vi "TurnToAngleController.vi"(0 "TargetAngle":dbl=600.0, 1 "MaxVel":dbl=80.0, 3 "MaxAccel":dbl=150.0, 5 "Robot":T1={"Angle"=548.1299999999924, "Angular vel"=0.49263510517714687, "Left Distance"=26.0882735, "Left vel"=0.0, "Right Distance"=-234.57467250000002, "Right vel"=0.0}, 9 "Gains":T2={"Gains"={"FFV"=0.0061, "FFA"=0.0024, "Vel PID"={"P"=0.0, "I"=0.0, "D"=0.0}}, "Pos PID"={"P"=0.0, "I"=0.0, "D"=0.0}, "MinVoltage"=0.25, "Effective Trackwidth"=30.0, "Effective Trackwidth CCW"=30.0} {"Pos PID"."D" format="%.3f"; "Pos PID"."I" format="%.3f"; "Pos PID"."P" format="%.3f"; "Gains"."Vel PID"."D" format="%.3f"; "Gains"."Vel PID"."I" format="%.3f"; "Gains"."Vel PID"."P" format="%.3f"}, 11 "Reset":bool, 13 "GoSmallestDistance":bool) -> (4 "LeftPower":dbl=0.25, 6 "RightPower":dbl=-0.25, 8 "Encoder Distance":cluster{"Output":dbl, "dx/dt":dbl}(graph)={"Output"=52.36486996421861, "dx/dt"=26.0882735}, 10 "Delay":dbl=20.0, 12 "Angle":cluster{"Distance":dbl, "CurrentAngle":dbl}(graph)={"Distance"=-120.0, "CurrentAngle"=-171.87000000000762}, 14 "VelGraph":cluster{"Output":dbl, "dx/dt":dbl}(graph), 15 "Done":bool)   [LabVIEW 2018]
uses:
  <vilib>/addons/control/pid/pid.llb/PID (DBL).vi
  <vilib>/addons/control/pid/NI_PID_pid.lvlib
panel:
  in  "Target Vel":dbl
  out "Power":dbl(graph)=0.25
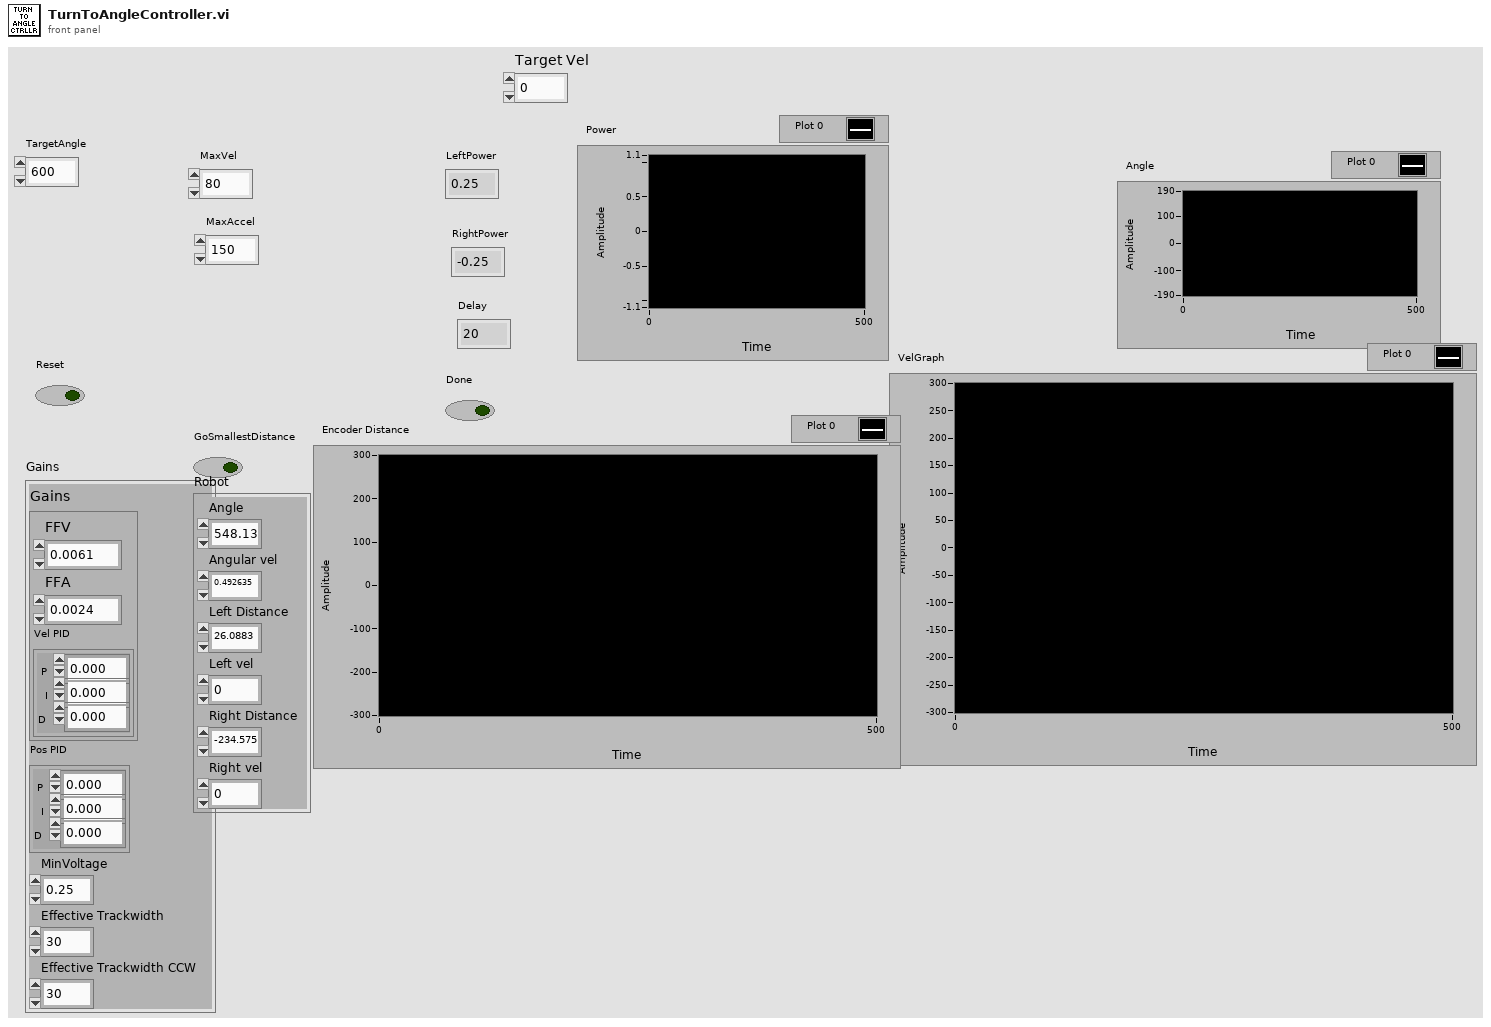
[diagram p1: front panel]
types:
  T1 = cluster{"Angle":dbl, "Angular vel":dbl, "Left Distance":dbl, "Left vel":dbl, "Right Distance":dbl, "Right vel":dbl}
  T2 = cluster{"Gains":cluster{"FFV":dbl, "FFA":dbl, "Vel PID":cluster{"P":dbl, "I":dbl, "D":dbl}}, "Pos PID":cluster{"P":dbl, "I":dbl, "D":dbl}, "MinVoltage":dbl, "Effective Trackwidth":dbl, "Effective Trackwidth CCW":dbl}
  T3 = cluster{"TargetPos":dbl, "InitalPos":dbl, "FinalVel":dbl, "IntitialVel":dbl, "MaxVel":dbl, "MaxAccel":dbl}
  T4 = cluster{"Smallest A to B":dbl, "Smallest A to B":dbl}
  T5 = cluster{"Smallest A to B":dbl, "Left Distance":dbl}
  T6 = cluster{"FFV":dbl, "FFA":dbl, "Vel PID":cluster{"P":dbl, "I":dbl, "D":dbl}}
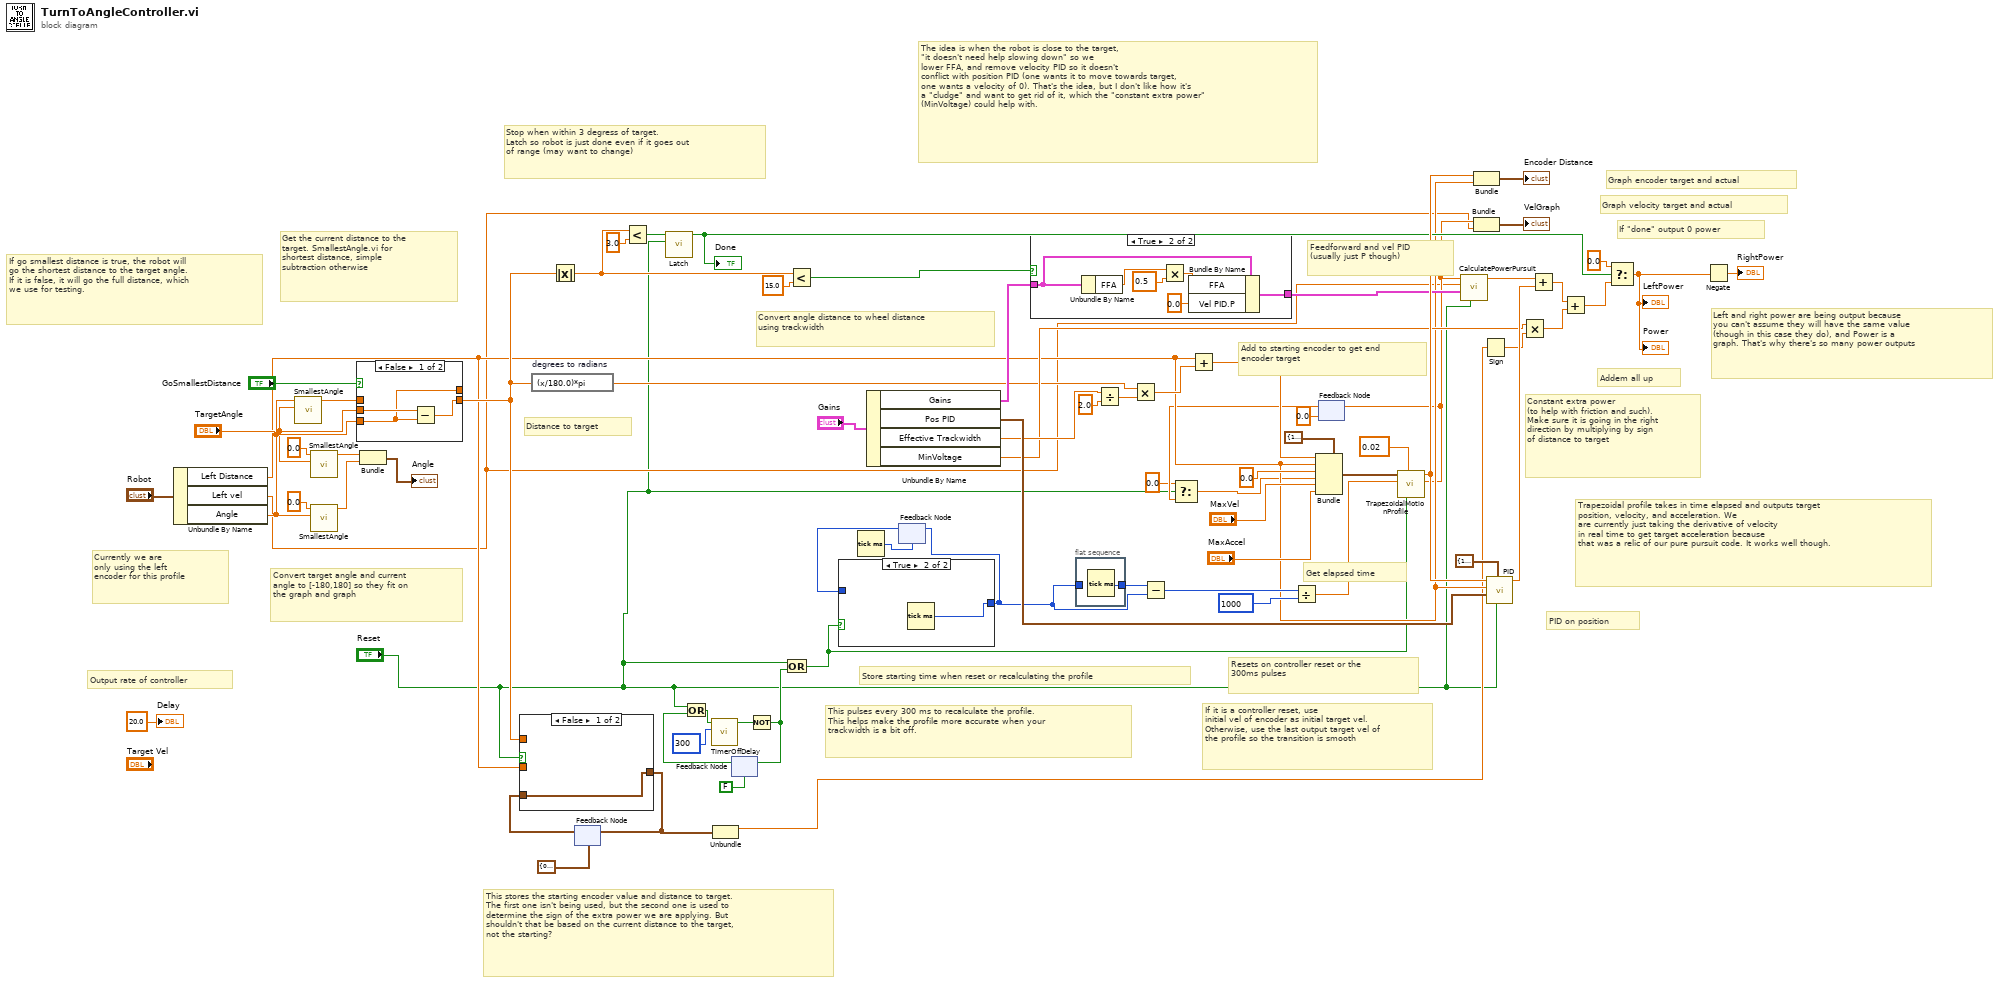
[diagram p0: block diagram]
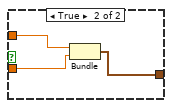
[diagram p2: hidden frame]
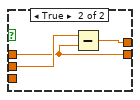
[diagram p4: hidden frame]
diagram:
  # "Currently we are\nonly using the left\nencoder for this profile"
  # "Output rate of controller"
  # "Addem all up"
  # "Left and right power are being output because\nyou can't assume they will have the same value\n(though in this case they do), and Power is a\ngraph. That's why there's so many power outputs"
  # "If \"done\" output 0 power"
  # "Graph velocity target and actual"
  # "Graph encoder target and actual"
  # "Feedforward and vel PID\n(usually just P though)"
  # "If it is a controller reset, use\ninitial vel of encoder as initial target vel.\nOtherwise, use the last output target vel of\nthe profile so the transition is smooth"
  # "Resets on controller reset or the \n300ms pulses"
  # "Trapezoidal profile takes in time elapsed and outputs target\nposition, velocity, and acceleration. We\nare currently just taking the derivative of velocity\nin real time to get target acceleration because\nthat was a relic of our pure pursuit code. It works well though."
  # "The idea is when the robot is close to the target,\n\"it doesn't need help slowing down\" so we\nlower FFA, and remove velocity PID so it doesn't\nconflict with position PID (one wants it to move towards target,\none wants a velocity of 0). That's the idea, but I don't like how it's\na \"cludge\" and want to get rid of it, which the \"constant extra power\"\n(MinVoltage) could help with."
  # "Add to starting encoder to get end\nencoder target"
  # "Convert angle distance to wheel distance\nusing trackwidth"
  # "Constant extra power\n(to help with friction and such).\nMake sure it is going in the right\ndirection by multiplying by sign\nof distance to target"
  # "PID on position"
  # "Get elapsed time"
  # "Store starting time when reset or recalculating the profile"
  # "This pulses every 300 ms to recalculate the profile.\nThis helps make the profile more accurate when your\ntrackwidth is a bit off."
  # "This stores the starting encoder value and distance to target.\nThe first one isn't being used, but the second one is used to\ndetermine the sign of the extra power we are applying. But\nshouldn't that be based on the current distance to the target,\nnot the starting?"
  # "Stop when within 3 degress of target.\nLatch so robot is just done even if it goes out\nof range (may want to change)"
  # "Get the current distance to the\ntarget. SmallestAngle.vi for \nshortest distance, simple\nsubtraction otherwise"
  # "If go smallest distance is true, the robot will\ngo the shortest distance to the target angle.\nIf it is false, it will go the full distance, which\nwe use for testing."
  # "Convert target angle and current\nangle to [-180,180] so they fit on\nthe graph and graph"
  # "Distance to target"
  n1 = Unbundle By Name("Robot") -> ("Left Distance"=w19:dbl, "Left vel"=w4:dbl, "Angle"=w53:dbl)
  n2 = call "SmallestAngle.vi"("Angle B"="TargetAngle", "Angle A"=w53) -> ("Smallest A to B"=w61:dbl)  [unwired: 9 in]
  n3 = call "SmallestAngle.vi"("Angle B"="TargetAngle", "Angle A"=0.0) -> ("Smallest A to B"=w51:dbl)  [unwired: 9 in]
  n4 = call "SmallestAngle.vi"("Angle B"=w53, "Angle A"=0.0) -> ("Smallest A to B"=w50:dbl)  [unwired: 9 in]
  n5 = case shown="False" "GoSmallestDistance" {
    tunnel: [w76 w80] -> _
    tunnel: "TargetAngle" -> [w77 w79]
    tunnel: w61 -> [_ w78]
    tunnel: [w75 w78] -> w20
    tunnel: w53 -> [w76 _]
    frame False {
      n6 = Subtract(x=w77, y=w76) -> (x-y=w75:dbl)
    }
    frame True {
      n7 = Subtract(x=w79, y=w78) -> (x-y=w80:dbl)
    }
  }
  n8 = Bundle("Smallest A to B"=w51, "Smallest A to B"=w50) -> (→"Angle":T4)  [unwired: 1 in]
  n9 = expression code="(x/180.0)*pi" "degrees to radians"(w20) -> (w18:dbl)
  n10 = Absolute Value(x=w20) -> (abs(x)=w31:dbl)
  n11 = feedback #1(cluster{"Angle":dbl, "Distance":dbl} {"Angle"=0.0, "Distance"=0.0}) -> (w35:cluster{"Angle":dbl, "Distance":dbl})
  n12 = case shown="False" "Reset" {
    tunnel: w20 -> [_ w84]
    tunnel: [w81 w83] -> w17
    tunnel: w35 -> [w81 _]
    tunnel: w19 -> [_ w82]
    frame False {
    }
    frame True {
      n13 = Bundle("Smallest A to B"=w84, "Left Distance"=w82) -> (w83:T5)  [unwired: 1 in]
    }
  }
  n14 = feedback-in #1(w17) -> ()
  n15 = Less?(x=w31, y=3.0) -> (x < y?=w57:bool)
  n16 = call "Latch.vi"("Reset"="Reset", "Input"=w57) -> ("Output"=w23:bool)  [unwired: 9 in]
  "Done" <- w23
  n17 = Unbundle(w17) -> ("Smallest A to B"=w16:dbl)  [unwired: 1 out]
  n18 = feedback #2(FALSE) -> (w11:bool)
  n19 = Or(x="Reset", y=w11) -> (x .or. y?=w12:bool)
  n20 = call "TimerOffDelay.vi"("Time Delay"=u32 300, "Input"=w12) -> ("Output"=w10:bool)  [unwired: 9 in]
  n21 = Not(x=w10) -> (.not. x?=w8:bool)
  n22 = feedback-in #2(w8) -> ()
  n23 = Or(x="Reset", y=w8) -> (x .or. y?=w14:bool)
  n24 = Less?(x=w31, y=15.0) -> (x < y?=w38:bool)
  n25 = Tick Count (ms)() -> (millisecond timer value=w36:u32)
  n26 = Unbundle By Name("Gains") -> ("Gains"=w39:T6, "Pos PID"=w45:cluster{"P":dbl, "I":dbl, "D":dbl}, "Effective Trackwidth"=w34:dbl, "MinVoltage"=w24:dbl)
  n27 = feedback #3(w36) -> (w37:u32)
  n28 = case shown="True" w14 {
    tunnel: [w85 w86] -> w29
    tunnel: w37 -> [w85 _]
    frame False {
    }
    frame True {
      n29 = Tick Count (ms)() -> (millisecond timer value=w86:u32)
    }
  }
  n30 = feedback-in #3(w29) -> ()
  n31 = case shown="True" w38 {
    tunnel: w39 -> [w87 w92]
    tunnel: [w87 w93] -> w22
    frame False {
    }
    frame True {
      n32 = Unbundle By Name(w92) -> ("FFA"=w91:dbl)
      n33 = Multiply(x=w91, y=0.5) -> (x*y=w89:dbl)
      n34 = Bundle By Name(cluster=w92, "FFA"=w89, "Vel PID.P"=0.0) -> (w93:T6)
    }
  }
  n35 = flat-sequence {
    tunnel: [w94] -> w67
    tunnel: w29 -> [_]
    frame #0 {
      n36 = Tick Count (ms)() -> (millisecond timer value=w94:u32)
    }
  }
  n37 = Divide(x=w34, y=2.0) -> (x/y=w48:dbl)
  n38 = Multiply(x=w18, y=w48) -> (x*y=w47:dbl)
  n39 = Subtract(x=w67, y=w29) -> (x-y=w66:u32)
  n40 = Add(x=w19, y=w47) -> (x+y=w46:dbl)
  n41 = Divide(x=w66, y=u32 1000) -> (x/y=w64:dbl)
  n42 = feedback #4(0.0 ("Velocity")) -> (w5:dbl)
  n43 = Select(t=0.0, s="Reset", f=w5) -> (s? t:f=w9:dbl)
  n44 = Bundle(cluster=T3 {"TargetPos"=10.0, "InitalPos"=0.0, "FinalVel"=0.0, "IntitialVel"=0.0, "MaxVel"=10.0, "MaxAccel"=10.0} ("Config"), "TargetPos"=w46, "InitalPos"=w19, "FinalVel"=0.0 ("IntitialVel"), "IntitialVel"=w9, "MaxVel"="MaxVel", "MaxAccel"="MaxAccel") -> (w68:T3)
  n45 = call "TrapezoidalMotionProfile.vi"("Initialize"=w14, "dt"=0.02, "Time"=w64, "Config"=w68) -> ("Velocity"=w7:dbl, "Distance"=w43:dbl)  [unwired: 4 in, 2 out]
  n46 = feedback-in #4(w7) -> ()
  n47 = call "CalculatePowerPursuit.vi"("Reset"="Reset", "Gains"=w22, "Vel"=w4, "Target Vel"=w7) -> ("Power"=w32:dbl)  [unwired: 7 in]
  n48 = Bundle("Distance"=w43, "Left Distance"=w19) -> (→"Encoder Distance":cluster{"Distance":dbl, "Left Distance":dbl})  [unwired: 1 in]
  n49 = Bundle("Velocity"=w7, "Left vel"=w4) -> (→"VelGraph":cluster{"Velocity":dbl, "Left vel":dbl})  [unwired: 1 in]
  n50 = Sign(1:w16) -> (0:w25:dbl)
  n51 = call-poly <vilib>:"PID.vi"("reinitialize? (F)"="Reset", "output range"=cluster{"output high":dbl, "output low":dbl} {"output high"=1.0, "output low"=-1.0}, "PID gains"=w45, "process variable"=w19, "setpoint"=w43) -> ("output"=w33:dbl)  [unwired: 5 in, 1 out]
  n52 = Multiply(x=w24, y=w25) -> (x*y=w26:dbl)
  n53 = Add(x=w32, y=w33) -> (x+y=w28:dbl)
  n54 = Add(x=w28, y=w26) -> (x+y=w27:dbl)
  n55 = Select(t=0.0, s=w23, f=w27) -> (s? t:f=w58:dbl)
  "LeftPower" <- w58
  "Power" <- w58
  n56 = Negate(x=w58) -> (-x=→"RightPower":dbl)
  "Delay" <- 20.0 ("Time Left")
